vi "FTW-Package-Request-Interpret.vi"(8 "error in":errorcluster, 11 "FTW Incoming Request":refnum<class "FTW-Package-IncomingRequest.lvclass">) -> (0 "error out":errorcluster, 1 "Request Body":string, 2 "Request Header":string, 3 "FTW Incoming Request out":refnum<class "FTW-Package-IncomingRequest.lvclass">)   [LabVIEW 2013, in "FTW-Package-IncomingRequest.lvclass"]
uses:
  FTW-Package-IncomingRequest.lvclass
  FTW-Package-IncomingRequest.lvclass/FTW-Package-IncomingRequest.ctl
  Base/FTW-Package.lvclass
panel:
  # "Inputs"
  # "Outputs"
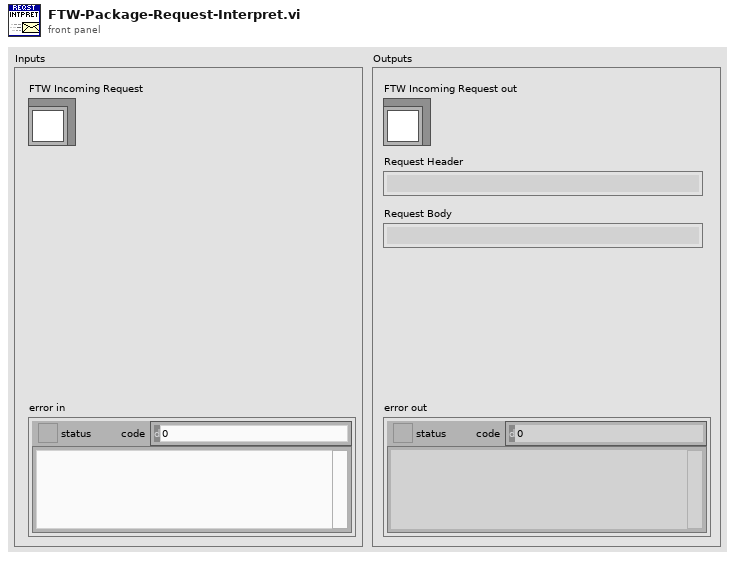
[diagram p1: front panel]
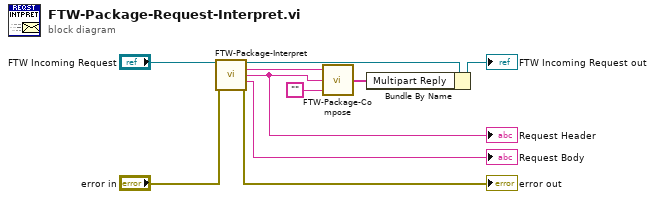
[diagram p0: block diagram]
diagram:
  n1 = call-dynamic "FTW-Package-Interpret.vi"("FTW Message"="FTW Incoming Request", "error in"="error in") -> ("FTW Message out"=w9:refnum<class "FTW-Package-IncomingRequest.lvclass">, "Sender Identity"=w5:string, "Message Header"=w3:string, "Message Body"=→"Request Body":string, "error out"=→"error out":errorcluster)  [unwired: 9 in]
  "Request Header" <- w3
  n2 = call "FTW-Package-Compose.vi"("Message Body"="", "Message Header"=w3, "Sender Identity"=w5) -> ("Multipart Message"=w4:string[])  [unwired: 1 in]
  n3 = Bundle By Name(cluster=w9, "Multipart Reply"=w4) -> (→"FTW Incoming Request out":refnum<class "FTW-Package-IncomingRequest.lvclass">)
